vi "AI Mean.vi"(7 "Samples to Avg":i32, 8 "Error IN":errorcluster, 11 "Serial Number":i32) -> (0 "Error OUT":errorcluster, 3 "Avg Data":dbl[](array[numeric]))   [LabVIEW 2010]
uses:
  <vilib>/Analysis/NI_AALBase.lvlib
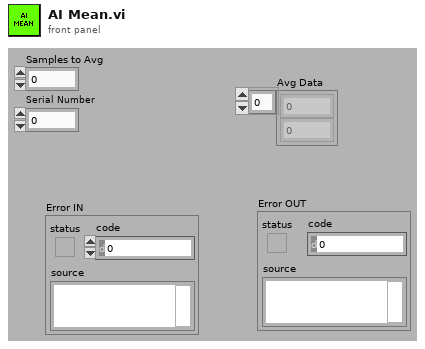
[diagram p1: front panel]
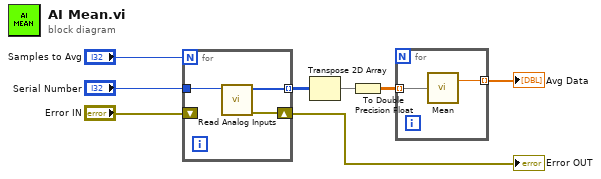
[diagram p0: block diagram]
diagram:
  n1 = for {
    N: "Samples to Avg" -> [_]
    tunnel: "Serial Number" -> [w11]
    tunnel: [w10] -> w6 mode=indexing
    shift-right: [w9] -> w2
    shift-left: "Error IN" -> [_]
    n2 = call <userlib>:"Read Analog Inputs.vi"("Serial Number"=w11) -> ("Error OUT"=w9:errorcluster, "Values"=w10:i32[])  [unwired: 9 in]
  }
  "Error OUT" <- w2
  n3 = Transpose 2D Array(2D array=w6) -> (transposed array=w5:i32[][])
  n4 = To Double Precision Float(number=w5) -> (double precision float=w4:dbl[][])
  n5 = for {
    tunnel: w4 -> [w13] mode=indexing
    tunnel: [w12] -> w1 mode=indexing
    n6 = call <vilib>:"Mean.vi"("X"=w13) -> ("mean"=w12:dbl)  [unwired: 1 out]
  }
  "Avg Data" <- w1
